vi "test_Expected Response Trigger.vi"(8 "error in (no error)":errorcluster, 11 "TestCase in":refnum<class "Expected Response Trigger test.lvclass">) -> (0 "error out":errorcluster, 3 "TestCase out":refnum<class "Expected Response Trigger test.lvclass">)   [LabVIEW 2017, in "Expected Response Trigger test.lvclass"]
uses:
  Expected Response Trigger test.lvclass
  Libraries/SSH/Expected Response String Config.ctl
  <vilib>/addons/_JKI Toolkits/VI Tester/TestCase.llb/TestCase.lvclass
  Libraries/SSH/SSH.lvlib
  C:/Program Files (x86)/National Instruments/LabVIEW 2017/vi.lib/addons/_JKI Toolkits/VI Tester/TestCase.llb/TestCase.lvclass
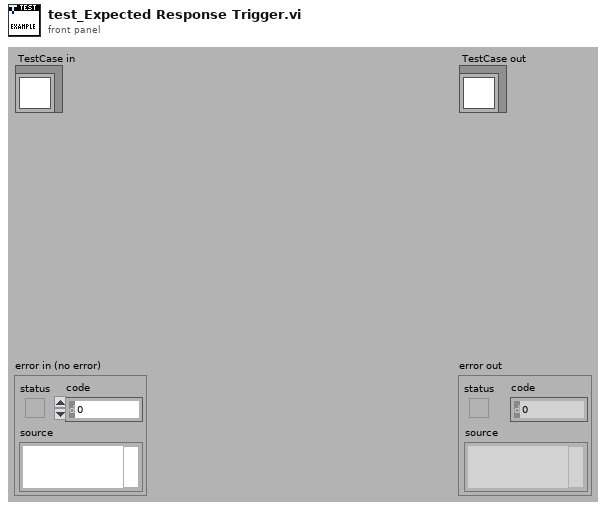
[diagram p1: front panel]
types:
  T1 = typedef "SSH.lvlib/Expected Response String Config.ctl" = cluster{"Expected Response":string, "Search Start Point":enum16{"From Start", "From End"}, "Instance Count":i32}
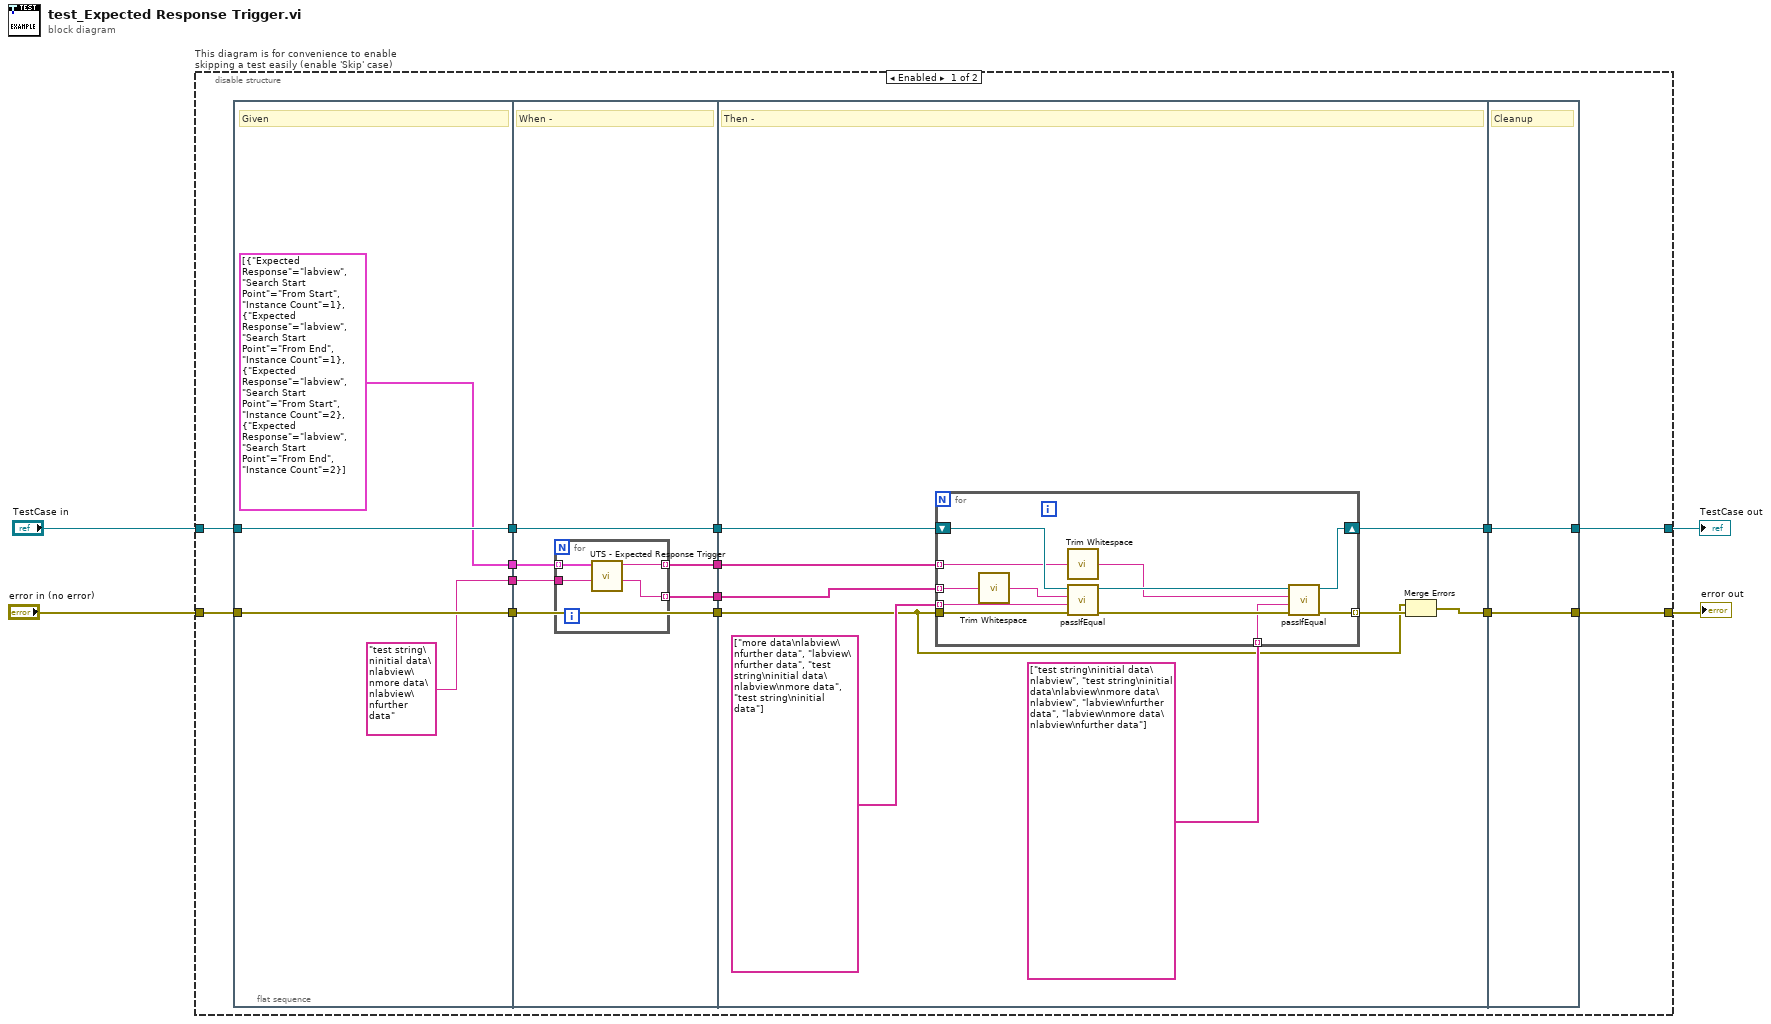
[diagram p0: block diagram]
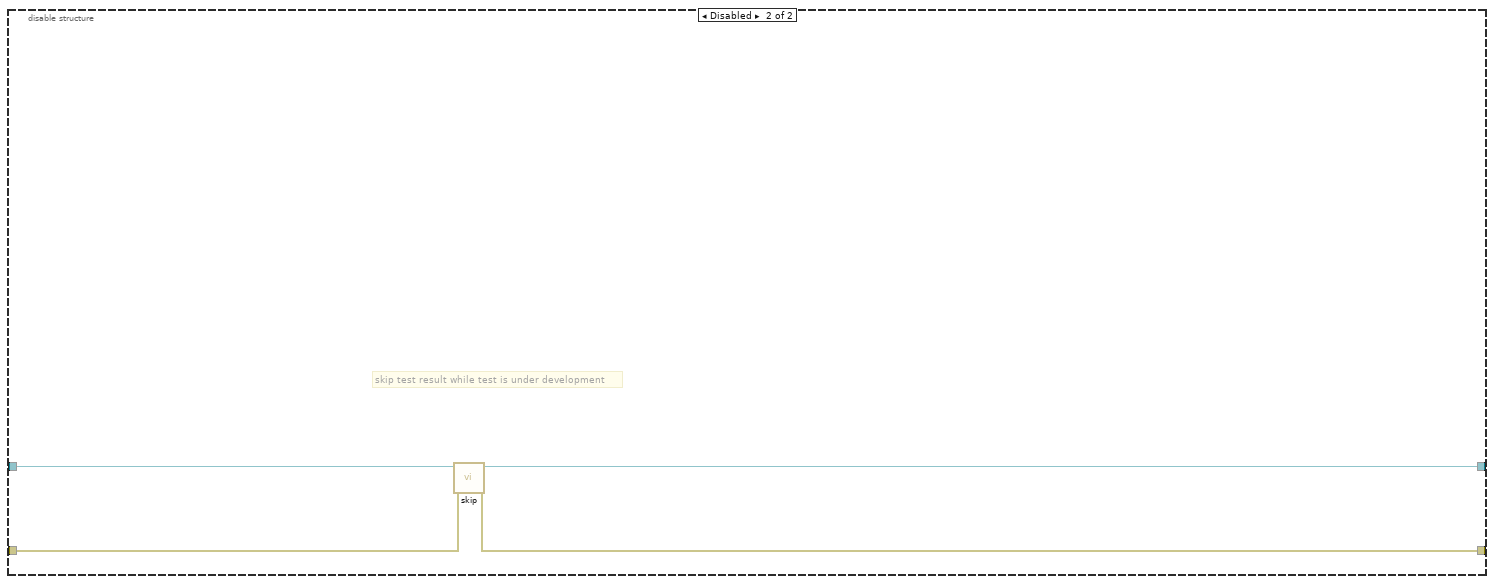
[diagram p2: hidden frame]
diagram:
  n1 = disable-structure "This diagram is for convenience to enable skipping a test easily (enable 'Skip' case)" shown="Enabled" {
    disable-tunnel: "TestCase in" -> [w11 w59]
    disable-tunnel: [w10 w57] -> w1
    disable-tunnel: [w9 w58] -> w3
    disable-tunnel: "error in (no error)" -> [w12 w56]
    frame Enabled {
      n2 = flat-sequence {
        tunnel: w12 -> [w21]
        tunnel: w11 -> [w22]
        tunnel: [w22] -> w18
        tunnel: [w21] -> w17
        tunnel: [T1[] [{"Expected Response"="labview", "Search Start Point"=enum."From Start", "Instance Count"=1}, {"Expected Response"="labview", "Search Start Point"=enum."From End", "Instance Count"=1}, {"Expected Response"="labview", "Search Start Point"=enum."From Start", "Instance Count"=2}, {"Expected Response"="labview", "Search Start Point"=enum."From End", "Instance Count"=2}] ("Expected Response")] -> w8
        tunnel: ["test string\ninitial data\nlabview\nmore data\nlabview\nfurther data" ("String Buffer in")] -> w7
        tunnel: [w28] -> w16
        tunnel: [w27] -> w15
        tunnel: w18 -> [w28]
        tunnel: w17 -> [w27]
        tunnel: w8 -> [w26]
        tunnel: w7 -> [w25]
        tunnel: [w24] -> w6
        tunnel: [w23] -> w5
        tunnel: [w41] -> w14
        tunnel: [w34] -> w13
        tunnel: w16 -> [w38]
        tunnel: w15 -> [w33]
        tunnel: w6 -> [w39]
        tunnel: w5 -> [w37]
        tunnel: [w54] -> w9
        tunnel: [w55] -> w10
        tunnel: w14 -> [w55]
        tunnel: w13 -> [w54]
        frame #0 {
          # "Given"
        }
        frame #1 {
          # "When -"
          n3 = for {
            tunnel: w26 -> [w32] mode=indexing
            tunnel: [w30] -> w24 mode=indexing
            tunnel: w25 -> [w31]
            tunnel: [w29] -> w23 mode=indexing
            n4 = call "UTS - Expected Response Trigger.vi"("String Buffer in"=w31, "Expected Response"=w32) -> ("String Buffer out"=w29:string, "Response"=w30:string)  [unwired: 7 in, 1 out]
          }
        }
        frame #2 {
          # "Then -"
          n5 = for {
            tunnel: w39 -> [w47] mode=indexing
            tunnel: w37 -> [w46] mode=indexing
            tunnel: string[] ["more data\nlabview\nfurther data", "labview\nfurther data", "test string\ninitial data\nlabview\nmore data", "test string\ninitial data"] ("String Buffer in") -> [w45] mode=indexing
            tunnel: string[] ["test string\ninitial data\nlabview", "test string\ninitial data\nlabview\nmore data\nlabview", "labview\nfurther data", "labview\nmore data\nlabview\nfurther data"] ("String Buffer in") -> [w44] mode=indexing
            shift-right: [w53] -> w41
            shift-left: w38 -> [w49]
            tunnel: w33 -> [w52]
            tunnel: [w51] -> w40 mode=indexing
            n6 = call <vilib>:"Trim Whitespace.vi"("string"=w46) -> ("trimmed string"=w43:string)  [unwired: 1 in]
            n7 = call <vilib>:"Trim Whitespace.vi"("string"=w47) -> ("trimmed string"=w42:string)  [unwired: 1 in]
            n8 = call-dynamic "passIfEqual.vi"("error in (no error)"=w52, "y"=w45, "x"=w43, "TestCase in"=w49) -> ("error out"=w50:errorcluster, "TestCase out"=w48:refnum<class "Expected Response Trigger test.lvclass">)  [unwired: 6 in]
            n9 = call-dynamic "passIfEqual.vi"("error in (no error)"=w50, "y"=w44, "x"=w42, "TestCase in"=w48) -> ("error out"=w51:errorcluster, "TestCase out"=w53:refnum<class "Expected Response Trigger test.lvclass">)  [unwired: 6 in]
          }
          n10 = Merge Errors(w33, w40) -> (w34:errorcluster)
        }
        frame #3 {
          # "Cleanup"
        }
      }
    }
    frame Disabled {
      # "skip test result while test is under development"
      n11 = call <vilib>:"skip.vi"("error in (no error)"=w56, "TestCase in"=w59) -> ("error out"=w58:errorcluster, "TestCase out"=w57:refnum<class "Expected Response Trigger test.lvclass">)  [unwired: 8 in]
    }
  }
  "error out" <- w3
  "TestCase out" <- w1
